vi "PH_Beckhoff-16BB.declare digital InputTags.vi"(2 "Racktype":string="N/A", 3 "Digital Inputs to be inverted [#s separated by ::]":string, 4 "Instance Name":string="<Instance Name>") -> (0 "Digital Inputs":T1, 1 "Description":string)   [LabVIEW 2014, in "PH_Beckhoff-16BB.lvlib"]
uses:
  PH_Beckhoff-16BB.lvlib
  PH_Beckhoff/PH_Beckhoff.Digital Inputs.ctl
  PH_Beckhoff-16BB.PA Chiller Tags.ctl
  PH_Beckhoff/PH_Beckhoff.lvlib
  PH_Beckhoff_Common/PH_Beckhoff_Common.lvlib
panel:
  out "Right Size?":bool
  # "Let this VI run to check the size!"
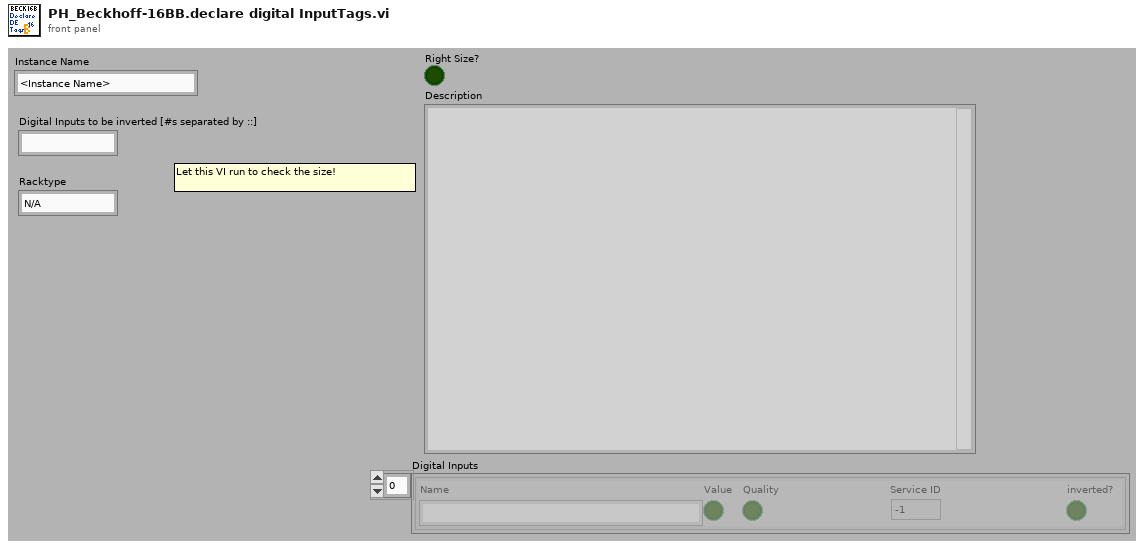
[diagram p1: front panel]
types:
  T1 = typedef "PH_Beckhoff.lvlib/PH_Beckhoff.Digital Inputs.ctl" = cluster{"Name":string, "Value":bool, "Quality":bool, "Service ID":i32, "inverted?":bool}[]
  T2 = cluster{"Name":string, "Value":bool, "Quality":bool, "Service ID":i32, "inverted?":bool}
  T3 = typedef "PH_Beckhoff-16BB.lvlib/PH_Beckhoff-16BB.PA Chiller Tags.ctl" = enum16{"Flow-control", "High-temp", "Conductivity", "Niveau", "Status"}
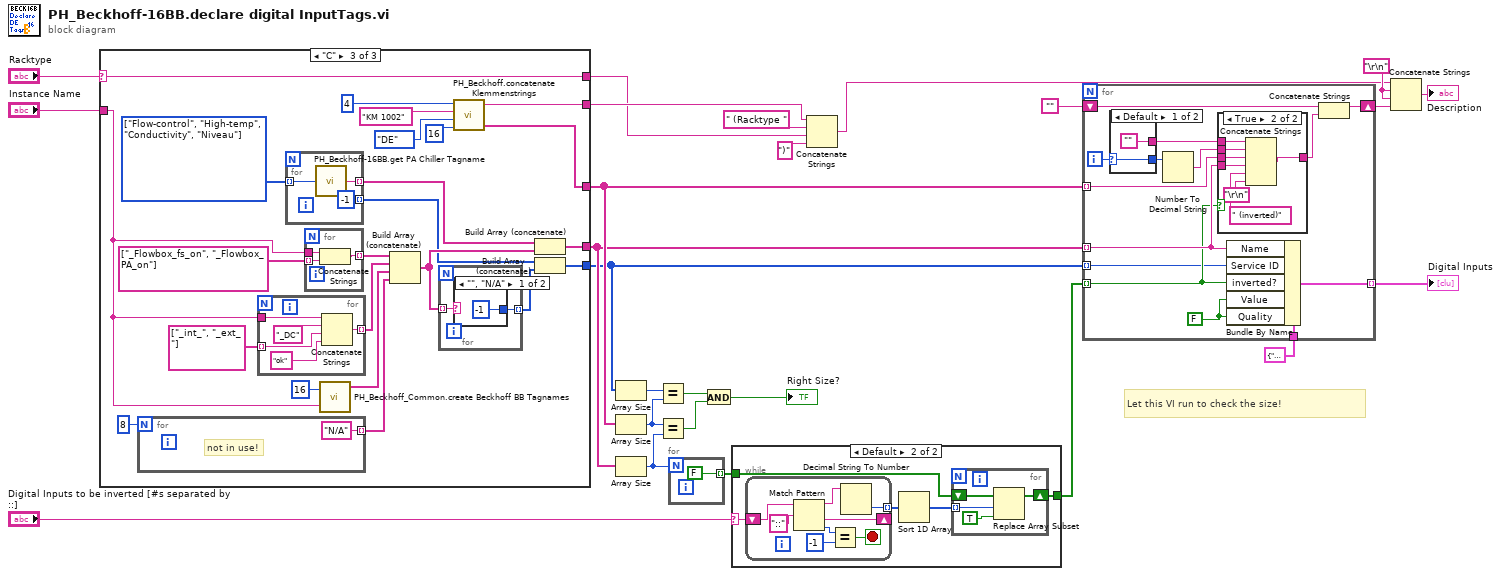
[diagram p0: block diagram]
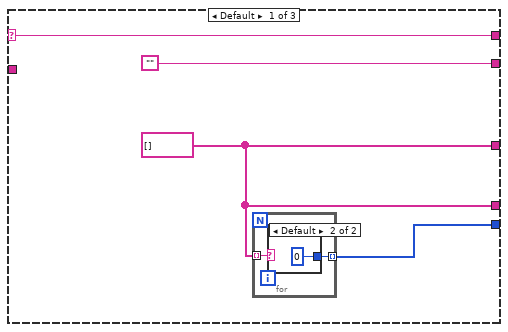
[diagram p2: hidden frame]
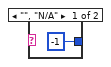
[diagram p3: hidden frame]
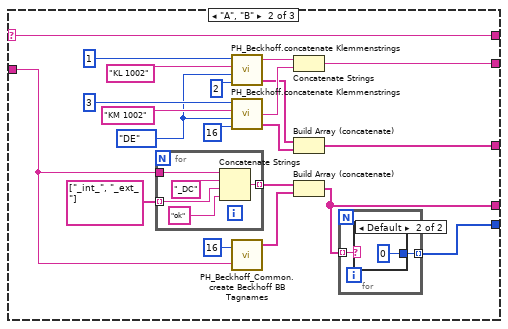
[diagram p4: hidden frame]
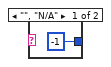
[diagram p5: hidden frame]
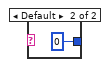
[diagram p6: hidden frame]
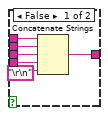
[diagram p8: hidden frame]
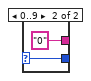
[diagram p9: hidden frame]
diagram:
  w25 = "\r\n"
  # "Let this VI run to check the size!"
  n1 = case shown="\"C\"" "Racktype" {
    selector: "Racktype" -> [w28 w39 w80]
    tunnel: "Instance Name" -> [_ w38 w72]
    tunnel: ["" w46 w74] -> w13
    tunnel: [w27 w35 w70] -> w9
    tunnel: [w27 w40 w79] -> w19
    tunnel: [w28 w39 w80] -> w12
    tunnel: [w26 w34 w65] -> w6
    frame Default {
      w27 = string[] []
      n2 = for {
        tunnel: w27 -> [w31] mode=indexing
        tunnel: [w30] -> w26 mode=indexing
        n3 = case shown="Default" w31 {
          tunnel: [-1 0] -> w30
          frame "", "N/A" {
          }
          frame Default {
          }
        }
      }
    }
    frame "A", "B" {
      w42 = enum16{"AE", "AA", "DE", "DA"}."DE" ("Type")
      n4 = for {
        tunnel: w38 -> [w63]
        tunnel: string[] ["_int_", "_ext_"] -> [w60] mode=indexing
        tunnel: [w62] -> w51 mode=indexing
        n5 = Concatenate Strings(w63, "_DC" ("string"), w60, "ok" ("string")) -> (w62:string)
      }
      n6 = call "PH_Beckhoff.concatenate Klemmenstrings.vi"("# of In- or Outputs"=2, "Type"=w42, "Klemmenname"="KL 1002", "Quantity"=1) -> ("concatenated string array"=w45:string[], "\"<Type>: <Quantity> x <Klemmenname>\""=w48:string)  [unwired: 1 out]
      n7 = call "PH_Beckhoff.concatenate Klemmenstrings.vi"("# of In- or Outputs"=16, "Type"=w42, "Klemmenname"="KM 1002", "Quantity"=3 ("size(s)")) -> ("concatenated string array"=w44:string[], "\"and <Quantity> x <Klemmenname>\""=w47:string)  [unwired: 1 out]
      n8 = call "PH_Beckhoff_Common.create Beckhoff BB Tagnames.vi"("#"=16, "Instance Name"=w38) -> ("Input Tags"=w36:string[])  [unwired: 2 out]
      n9 = Concatenate Strings(w48, w47) -> (w46:string)
      n10 = Build Array (concatenate)(w45, w44) -> (w40:string[])
      n11 = Build Array (concatenate)(w51, w36) -> (w35:string[])
      n12 = for {
        tunnel: w35 -> [w56] mode=indexing
        tunnel: [w55] -> w34 mode=indexing
        n13 = case shown="Default" w56 {
          tunnel: [-1 0] -> w55
          frame "", "N/A" {
          }
          frame Default {
          }
        }
      }
    }
    frame "C" {
      w68 = T3[] [enum."Flow-control", enum."High-temp", enum."Conductivity", enum."Niveau"] items=["Flow-control", "High-temp", "Conductivity", "Niveau", "Status"]
      n14 = for {
        N: 8 -> [_]
        tunnel: ["N/A" ("string")] -> w77 mode=indexing
        # "not in use!"
      }
      n15 = for {
        tunnel: w72 -> [w102]
        tunnel: string[] ["_int_", "_ext_"] -> [w99] mode=indexing
        tunnel: [w101] -> w83 mode=indexing
        n16 = Concatenate Strings(w102, "_DC" ("string"), w99, "ok" ("string")) -> (w101:string)
      }
      n17 = for {
        tunnel: [w93] -> w69 mode=indexing
        tunnel: w68 -> [w92] mode=indexing
        tunnel: [-1] -> w64 mode=indexing
        n18 = call "PH_Beckhoff-16BB.get PA Chiller Tagname.vi"("PA Chiller Tag"=w92) -> ("PA Chiller Tagname"=w93:string)
      }
      n19 = for {
        tunnel: w72 -> [w96]
        tunnel: string[] ["_Flowbox_fs_on", "_Flowbox_PA_on"] -> [w94] mode=indexing
        tunnel: [w95] -> w75 mode=indexing
        n20 = Concatenate Strings(w96, w94) -> (w95:string)
      }
      n21 = call "PH_Beckhoff_Common.create Beckhoff BB Tagnames.vi"("#"=16, "Instance Name"=w72) -> ("Input Tags"=w71:string[])  [unwired: 2 out]
      n22 = Build Array (concatenate)(w75, w83, w71, w77) -> (w67:string[])
      n23 = for {
        tunnel: w67 -> [w88] mode=indexing
        tunnel: [w87] -> w66 mode=indexing
        n24 = case shown="\"\", \"N/A\"" w88 {
          tunnel: [-1 0] -> w87
          frame "", "N/A" {
          }
          frame Default {
          }
        }
      }
      n25 = call "PH_Beckhoff.concatenate Klemmenstrings.vi"("# of In- or Outputs"=16, "Type"=enum16{"AE", "AA", "DE", "DA"}."DE", "Klemmenname"="KM 1002", "Quantity"=4 ("size(s)")) -> ("concatenated string array"=w79:string[], "\"<Type>: <Quantity> x <Klemmenname>\""=w74:string)  [unwired: 1 out]
      n26 = Build Array (concatenate)(w69, w67) -> (w70:string[])
      n27 = Build Array (concatenate)(w64, w66) -> (w65:i32[])
    }
  }
  n28 = Array Size(array=w6) -> (size(s)=w5:i32)
  n29 = Array Size(array=w19) -> (size(s)=w4:i32)
  n30 = Array Size(array=w9) -> (size(s)=w10:i32)
  n31 = Equal?(x=w5, y=w4) -> (x = y?=w1:bool)
  n32 = Equal?(x=w4, y=w10) -> (x = y?=w2:bool)
  n33 = for {
    N: w10 -> [_]
    tunnel: [FALSE] -> w22 mode=indexing
  }
  n34 = And(x=w1, y=w2) -> (x .and. y?=→"Right Size?":bool)
  n35 = case shown="Default" "Digital Inputs to be inverted [#s separated by ::]" {
    selector: "Digital Inputs to be inverted [#s separated by ::]" -> [_ w109]
    tunnel: w22 -> [w104 w106]
    tunnel: [w104 w105] -> w11
    frame "", "N/A" {
    }
    frame Default {
      n36 = while {
        shift-right: [w116] -> _
        shift-left: w109 -> [w121]
        tunnel: [w114] -> w108 mode=indexing
        stop <- w117 stop-if-true
        n37 = Match Pattern(string=w121, regular expression="::") -> (before substring=w115:string, after substring=w116:string, offset past match=w119:i32)  [unwired: 1 in, 1 out]
        n38 = Equal?(x=w119, y=-1) -> (x = y?=w117:bool)
        n39 = Decimal String To Number(string=w115) -> (number=w114:i32)  [unwired: 2 in, 1 out]
      }
      n40 = Sort 1D Array(array=w108) -> (sorted array=w107:i32[])
      n41 = for {
        tunnel: w107 -> [w111] mode=indexing
        shift-right: [w112] -> w105
        shift-left: w106 -> [w113]
        n42 = Replace Array Subset(array=w113, new element=TRUE ("new element/subarray"), index=w111) -> (w112:bool[])
      }
    }
  }
  n43 = Concatenate Strings(w13, " (Racktype " ("string"), w12, ")" ("string")) -> (w14:string)
  n44 = for {
    tunnel: w9 -> [w126] mode=indexing
    tunnel: w19 -> [w131] mode=indexing
    shift-right: [w129] -> w20
    shift-left: "" -> [w128]
    tunnel: w11 -> [w125] mode=indexing
    tunnel: T2 {"Name"="", "Value"=FALSE, "Quality"=FALSE, "Service ID"=0, "inverted?"=FALSE} ("Digital Input Value") -> [w127]
    tunnel: [w123] -> w7 mode=indexing
    tunnel: w6 -> [w122] mode=indexing
    i -> [w135]
    w124 = FALSE ("Quality")
    n45 = case shown="Default" w135 {
      selector: w135 -> [w149 w152]
      tunnel: [w149 w152] -> w134
      tunnel: ["" "0"] -> w133
      frame Default {
      }
      frame 0..9 {
      }
    }
    n46 = Number To Decimal String(number=w134) -> (decimal integer string=w132:string)  [unwired: 1 in]
    n47 = case shown="True" w125 {
      tunnel: w133 -> [w141 w148]
      tunnel: w132 -> [w140 w147]
      tunnel: w131 -> [w139 w146]
      tunnel: w126 -> [w138 w145]
      tunnel: [w136 w143] -> w130
      frame False {
        n48 = Concatenate Strings(w141, w140, w139, w138, "\r\n") -> (w136:string)
      }
      frame True {
        n49 = Concatenate Strings(w148, w147, w146, w145, " (inverted)", "\r\n") -> (w143:string)
      }
    }
    n50 = Bundle By Name(cluster=w127, "Name"=w126, "Service ID"=w122, "inverted?"=w125, "Value"=w124, "Quality"=w124) -> (w123:T2)
    n51 = Concatenate Strings(w128, w130) -> (w129:string)
  }
  "Digital Inputs" <- w7
  n52 = Concatenate Strings(w14, w25, w25, w20) -> (→"Description":string)
